vi "Extract2Dprojections-xy-zx-zy.vi"(7 "max plot":bool, 11 "zyx":u16[][][](array[numeric])) -> (1 "yx":u16[][](array[numeric]), 2 "zx":u16[][](array[numeric]), 3 "zy":u16[][](array[numeric]))   [LabVIEW 2024]
panel:
  out "x*y":i32
  in  "bg count":i32
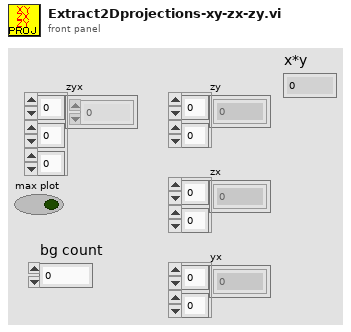
[diagram p1: front panel]
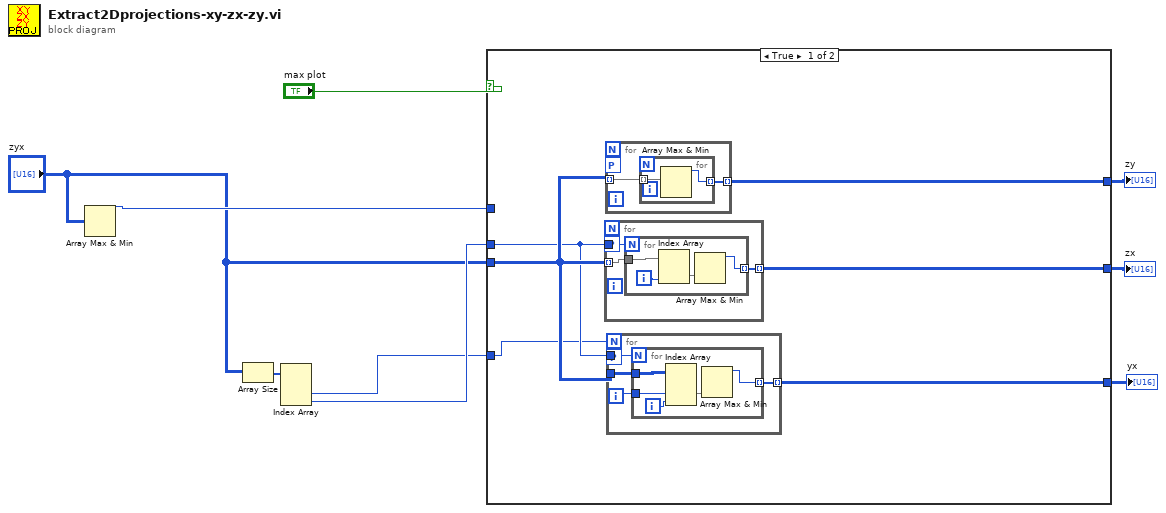
[diagram p0: block diagram]
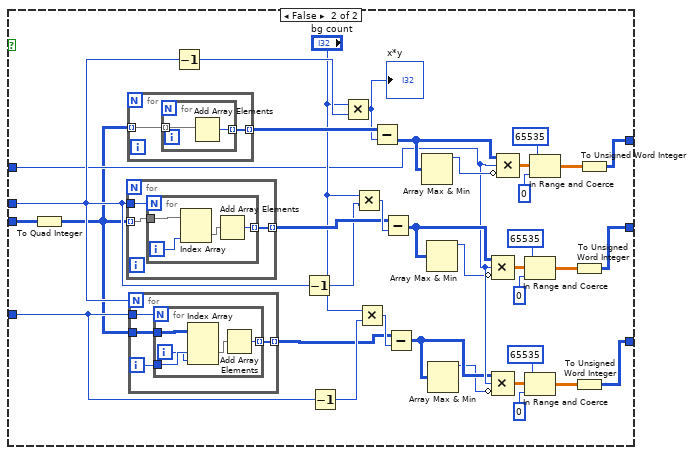
[diagram p2: hidden frame]
diagram:
  n1 = Array Max & Min(array="zyx") -> (max value=w2:u16)  [unwired: 3 out]
  n2 = Array Size(array="zyx") -> (size(s)=w4:i32[])
  n3 = Index Array(array=w4) -> (element #2=w5:i32, element #3=w6:i32)  [unwired: 3 in, 1 out]
  n4 = case shown="True" "max plot" {
    tunnel: [w12 w38] -> w9
    tunnel: [w15 w39] -> w8
    tunnel: [w14 w56] -> w7
    tunnel: w6 -> [w11 w64]
    tunnel: w5 -> [w10 w63]
    tunnel: "zyx" -> [w13 w71]
    tunnel: w2 -> [_ w43]
    frame True {
      n5 = for {
        tunnel: w13 -> [w27] mode=indexing
        tunnel: w11 -> [w26]
        tunnel: [w25] -> w15 mode=indexing
        workers-P: _ -> [_]
        n6 = for {
          N: w26 -> [_]
          tunnel: w27 -> [w31]
          tunnel: [w28] -> w25 mode=indexing
          i -> [w30]
          n7 = Index Array(array=w31, index (col)=w30) -> (element=w29:u16[])  [unwired: 1 in]
          n8 = Array Max & Min(array=w29) -> (max value=w28:u16)  [unwired: 3 out]
        }
      }
      n9 = for {
        tunnel: w13 -> [w33] mode=indexing
        tunnel: [w32] -> w14 mode=indexing
        workers-P: _ -> [_]
        n10 = for {
          tunnel: w33 -> [w35] mode=indexing
          tunnel: [w34] -> w32 mode=indexing
          n11 = Array Max & Min(array=w35) -> (max value=w34:u16)  [unwired: 3 out]
        }
      }
      n12 = for {
        N: w10 -> [_]
        tunnel: w13 -> [w19]
        tunnel: w11 -> [w18]
        tunnel: [w17] -> w12 mode=indexing
        workers-P: _ -> [_]
        i -> [w16]
        n13 = for {
          N: w18 -> [_]
          tunnel: w19 -> [w24]
          tunnel: [w22] -> w17 mode=indexing
          tunnel: w16 -> [w20]
          i -> [w21]
          n14 = Index Array(array=w24, index (dim 1)=w20, index (dim 2)=w21) -> (element=w23:u16[])  [unwired: 1 in]
          n15 = Array Max & Min(array=w23) -> (max value=w22:u16)  [unwired: 3 out]
        }
      }
    }
    frame False {
      n16 = To Quad Integer(1:w71) -> (0:w37:i64[][][])
      n17 = for {
        tunnel: w37 -> [w83] mode=indexing
        tunnel: w64 -> [w82]
        tunnel: [w81] -> w65 mode=indexing
        n18 = for {
          N: w82 -> [_]
          tunnel: w83 -> [w87]
          tunnel: [w84] -> w81 mode=indexing
          i -> [w86]
          n19 = Index Array(array=w87, index (col)=w86) -> (element=w85:i64[])  [unwired: 1 in]
          n20 = Add Array Elements(numeric array=w85) -> (sum=w84:i64)
        }
      }
      n21 = for {
        tunnel: w37 -> [w89] mode=indexing
        tunnel: [w88] -> w70 mode=indexing
        n22 = for {
          tunnel: w89 -> [w91] mode=indexing
          tunnel: [w90] -> w88 mode=indexing
          n23 = Add Array Elements(numeric array=w91) -> (sum=w90:i64)
        }
      }
      n24 = for {
        N: w64 -> [_]
        tunnel: w37 -> [w75]
        tunnel: w63 -> [w74]
        tunnel: [w73] -> w36 mode=indexing
        i -> [w72]
        n25 = for {
          N: w74 -> [_]
          tunnel: w75 -> [w80]
          tunnel: [w78] -> w73 mode=indexing
          tunnel: w72 -> [w77]
          i -> [w76]
          n26 = Index Array(array=w80, index (dim 1)=w77, index (dim 2)=w76) -> (element=w79:i64[])  [unwired: 1 in]
          n27 = Add Array Elements(numeric array=w79) -> (sum=w78:i64)
        }
      }
      n28 = Decrement(x=w64) -> (x-1=w69:i32)
      n29 = Decrement(x=w64) -> (x-1=w61:i32)
      n30 = Decrement(x=w63) -> (x-1=w60:i32)
      n31 = Multiply(x="bg count", y=w69) -> (x*y=w68:i32)
      "x*y" <- w68
      n32 = Multiply(x="bg count", y=w61) -> (x*y=w67:i32)
      n33 = Multiply(x="bg count", y=w60) -> (x*y=w66:i32)
      n34 = Subtract(x=w70, y=w68) -> (x-y=w59:i64[][])
      n35 = Subtract(x=w65, y=w67) -> (x-y=w44:i64[][])
      n36 = Subtract(x=w36, y=w66) -> (x-y=w42:i64[][])
      n37 = Array Max & Min(array=w59) -> (max value=w58:i64)  [unwired: 3 out]
      n38 = Array Max & Min(array=w44) -> (max value=w41:i64)  [unwired: 3 out]
      n39 = Array Max & Min(array=w42) -> (max value=w40:i64)  [unwired: 3 out]
      n40 = Compound Arithmetic op=MULTIPLY(w44, w43, invert w41) -> (w49:dbl[][])
      n41 = Compound Arithmetic op=MULTIPLY(w42, w43, invert w40) -> (w48:dbl[][])
      n42 = Compound Arithmetic op=MULTIPLY(w59, w43, invert w58) -> (w57:dbl[][])
      n43 = In Range and Coerce(upper limit=65535, x=w49, lower limit=0) -> (coerced(x)=w50:dbl[][])  [unwired: 1 out]
      n44 = In Range and Coerce(upper limit=65535, x=w48, lower limit=0) -> (coerced(x)=w47:dbl[][])  [unwired: 1 out]
      n45 = In Range and Coerce(upper limit=65535, x=w57, lower limit=0) -> (coerced(x)=w55:dbl[][])  [unwired: 1 out]
      n46 = To Unsigned Word Integer(number=w50) -> (unsigned 16bit integer=w39:u16[][])
      n47 = To Unsigned Word Integer(number=w47) -> (unsigned 16bit integer=w38:u16[][])
      n48 = To Unsigned Word Integer(number=w55) -> (unsigned 16bit integer=w56:u16[][])
    }
  }
  "yx" <- w9
  "zx" <- w8
  "zy" <- w7
